vi "add units.vi"(7 "Language":string, 9 "Array":dbl[](array[numeric]), 10 "Numeric":dbl, 11 "Label Text":string) -> (1 "Converted Array":dbl[](array[numeric]), 2 "Converted Numeric":dbl, 3 "unit in brackets":string, 4 "format string":string, 5 "unit":string)   [LabVIEW 2015]
panel:
  # "Et\tEntrance Tank\tformerly grit chamber\nAmp\tamplitude\tL\nB\tperpendicular distance between components (center to center)\tL\nE\tpipe roughness\tL\nFB\tFreeboard\tL\nH\theight (includes freeboard)\tL\nHL\thead loss\tL\nHW\tlocal water depth\tL\nID\tinner diameter\tL\nL\tlength\tL\nLoc\tLocations\tL\nND\tnominal diameter\tL\nOD\touter diameter\tL\nR\tRadius\tL\nS\tspace between components\tL\nT\tthickness\tL\nW\twidth\tL\nZ\televation relative to bottom of sed tank\tL\nZW\twater depth relative to bottom of sed tank\tL\nV\tvelocity\tL/T\nCP\tCollision Potential\tL^(2/3)\nA\tArea\tL^2\nNu\tkinematic viscosity\tL^2/T\nED\tenergy dissipation rate\tL^2/T^3\nVol\tvolume\tL^3\nQ\tflow\tL^3/T\nMW\tMolecular weight\tM\nC\tConcentration\tM/L^3\nRho\tDensity\tM/L^3\nAN\tangle\tradians\nTi\ttime\tT"
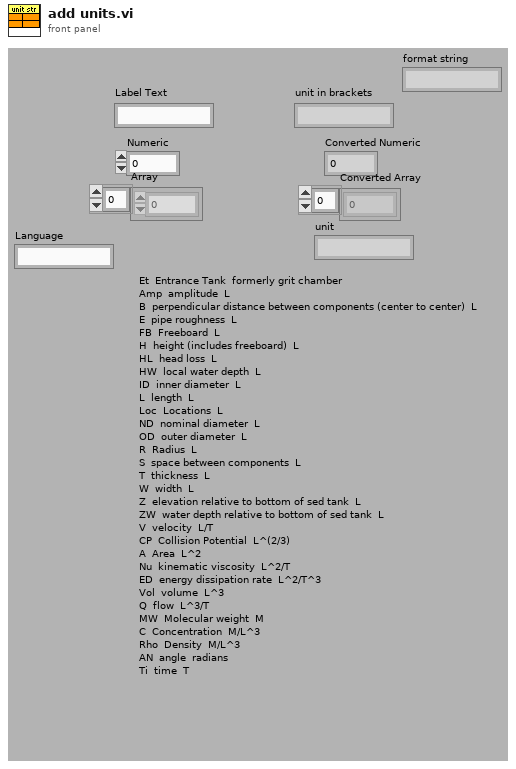
[diagram p1: front panel]
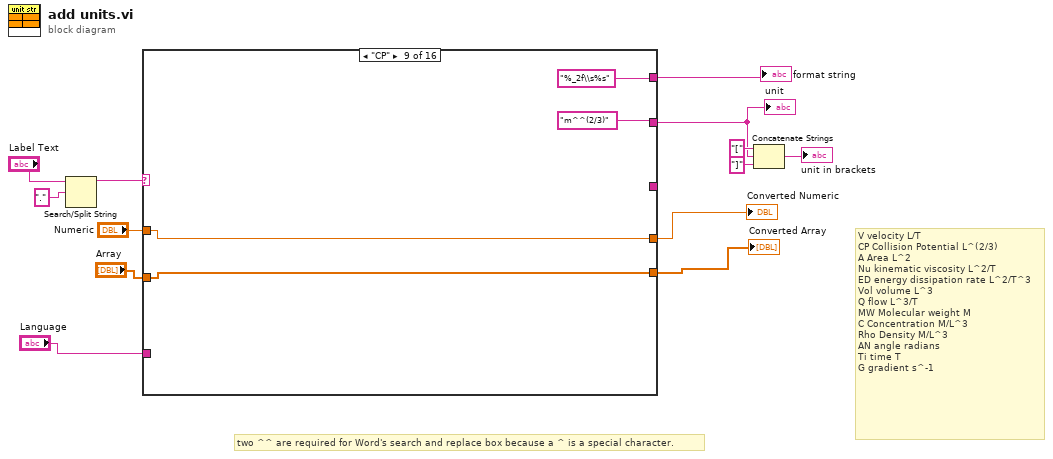
[diagram p0: block diagram]
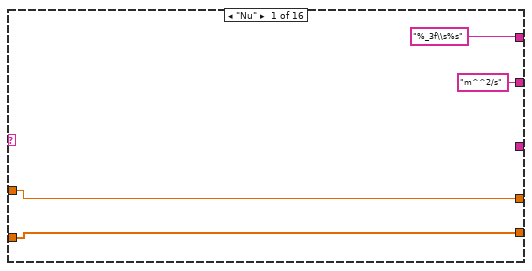
[diagram p2: hidden frame]
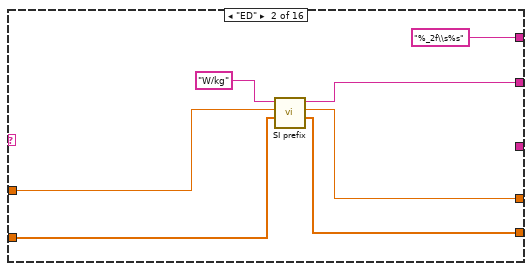
[diagram p3: hidden frame]
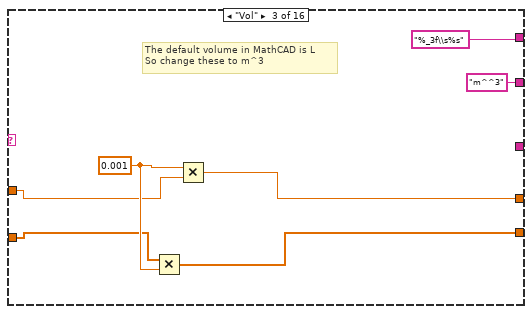
[diagram p4: hidden frame]
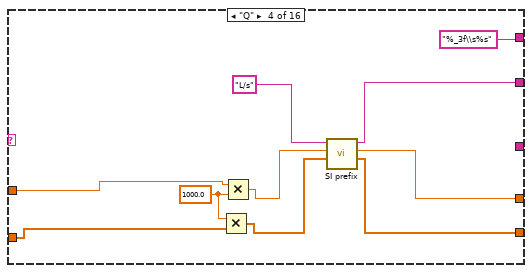
[diagram p5: hidden frame]
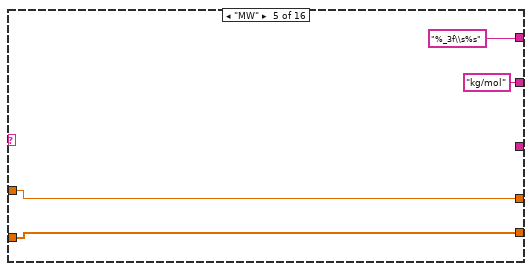
[diagram p6: hidden frame]
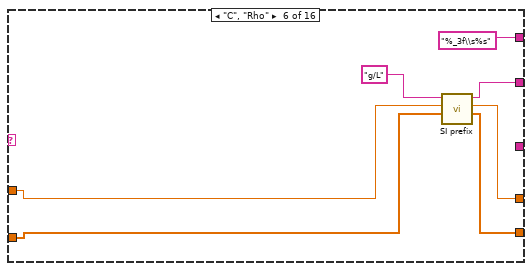
[diagram p7: hidden frame]
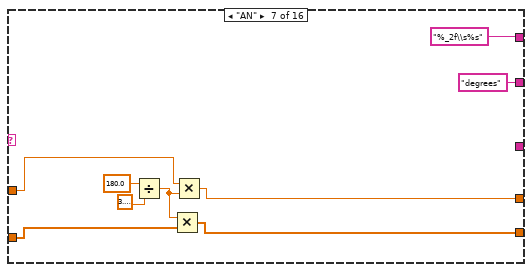
[diagram p8: hidden frame]
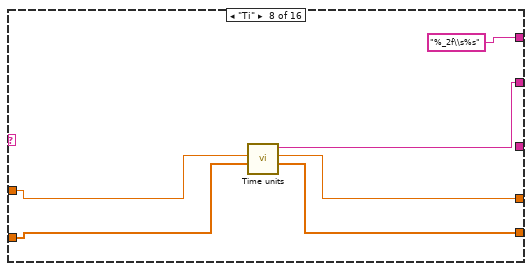
[diagram p9: hidden frame]
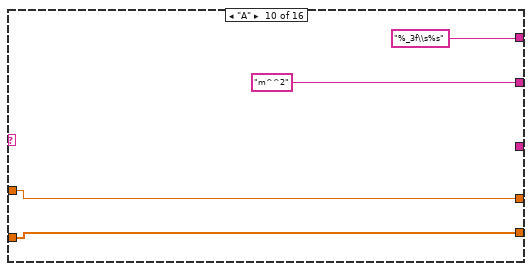
[diagram p10: hidden frame]
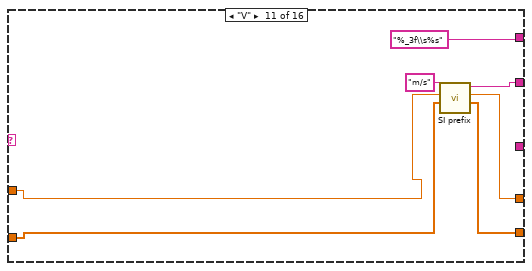
[diagram p11: hidden frame]
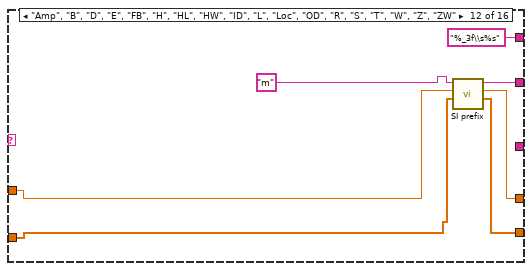
[diagram p12: hidden frame]
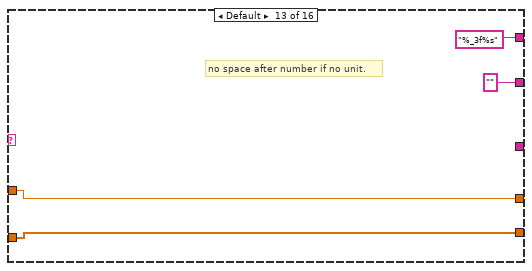
[diagram p13: hidden frame]
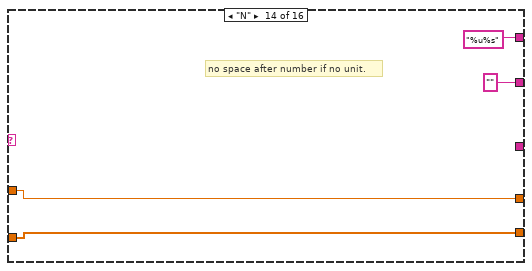
[diagram p14: hidden frame]
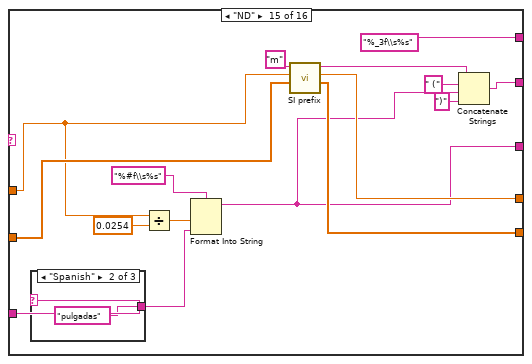
[diagram p15: hidden frame]
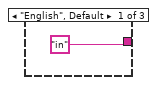
[diagram p16: hidden frame]
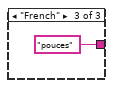
[diagram p17: hidden frame]
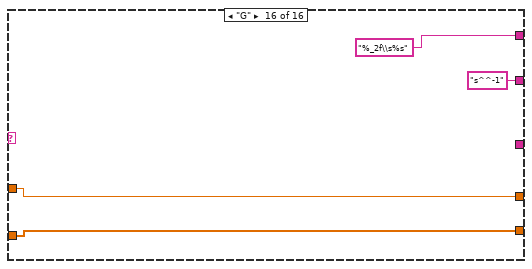
[diagram p18: hidden frame]
diagram:
  # "two ^^ are required for Word's search and replace box because a ^ is a special character."
  # "V\tvelocity\tL/T\nCP\tCollision Potential\tL^(2/3)\nA\tArea\tL^2\nNu\tkinematic viscosity\tL^2/T\nED\tenergy dissipation rate\tL^2/T^3\nVol\tvolume\tL^3\nQ\tflow\tL^3/T\nMW\tMolecular weight\tM\nC\tConcentration\tM/L^3\nRho\tDensity\tM/L^3\nAN\tangle\tradians\nTi\ttime\tT\nG gradient s^-1"
  n1 = Search/Split String(string="Label Text", search string/char (-)="." ("regular expression")) -> (substring before match=w11:string)  [unwired: 1 in, 2 out]
  n2 = case shown="\"CP\"" w11 {
    tunnel: ["m^^2/s" w22 "m^^3" w36 "kg/mol" w50 "degrees" w62 "m^^(2/3)" "m^^2" w80 w87 "" "" w103 "s^^-1" ("modified unit")] -> w4
    tunnel: "Numeric" -> [w16 w21 w28 w40 w44 w49 w57 w66 w70 w74 w77 w86 w92 w96 w109 w119]
    tunnel: "Array" -> [w15 w20 w26 w39 w43 w47 w56 w65 w69 w73 w79 w84 w91 w95 w112 w118]
    tunnel: [w15 w18 w25 w32 w43 w46 w54 w64 w69 w73 w78 w83 w91 w95 w111 w118] -> w2
    tunnel: [w16 w19 w27 w34 w44 w48 w55 w63 w70 w74 w76 w85 w92 w96 w110 w119] -> w3
    tunnel: ["%_3f\\s%s" "%_2f\\s%s" "%_3f\\s%s" "%_3f\\s%s" "%_3f\\s%s" "%_3f\\s%s" "%_2f\\s%s" "%_2f\\s%s" "%_2f\\s%s" "%_3f\\s%s" "%_3f\\s%s" "%_3f\\s%s" "%_3f%s" "%u%s" "%_3f\\s%s" "%_2f\\s%s"] -> w5
    tunnel: [_ _ _ _ _ _ _ _ _ _ _ _ _ _ w102 _] -> _
    tunnel: "Language" -> [_ _ _ _ _ _ _ _ _ _ _ _ _ _ w99 _]
    frame "Nu" {
    }
    frame "ED" {
      n3 = call "SI prefix.vi"("Array"=w20, "Numeric"=w21, "Unit"="W/kg") -> ("Scaled Array"=w18:dbl[], "Scaled Number"=w19:dbl, "modified unit"=w22:string)  [unwired: 6 in]
    }
    frame "Vol" {
      w29 = 0.001 ("x")
      # "The default volume in MathCAD is L\nSo change these to m^3"
      n4 = Multiply(x=w26, y=w29) -> (x*y=w25:dbl[])
      n5 = Multiply(x=w29, y=w28) -> (x*y=w27:dbl)
    }
    frame "Q" {
      w41 = 1000.0 ("y")
      n6 = Multiply(x=w41, y=w39) -> (x*y=w33:dbl[])
      n7 = Multiply(x=w40, y=w41) -> (x*y=w35:dbl)
      n8 = call "SI prefix.vi"("Array"=w33, "Numeric"=w35, "Unit"="L/s") -> ("Scaled Array"=w32:dbl[], "Scaled Number"=w34:dbl, "modified unit"=w36:string)  [unwired: 6 in]
    }
    frame "MW" {
    }
    frame "C", "Rho" {
      n9 = call "SI prefix.vi"("Array"=w47, "Numeric"=w49, "Unit"="g/L") -> ("Scaled Array"=w46:dbl[], "Scaled Number"=w48:dbl, "modified unit"=w50:string)  [unwired: 6 in]
    }
    frame "AN" {
      n10 = Divide(x=180.0 ("y"), y=3.141592653589793) -> (x/y=w60:dbl)
      n11 = Multiply(x=w60, y=w56) -> (x*y=w54:dbl[])
      n12 = Multiply(x=w57, y=w60) -> (x*y=w55:dbl)
    }
    frame "Ti" {
      n13 = call "Time units.vi"("Array"=w65, "Numeric"=w66) -> ("Scaled Array"=w64:dbl[], "Scaled Number"=w63:dbl, "modified unit"=w62:string)  [unwired: 7 in]
    }
    frame "CP" {
    }
    frame "A" {
    }
    frame "V" {
      n14 = call "SI prefix.vi"("Array"=w79, "Numeric"=w77, "Unit"="m/s") -> ("Scaled Array"=w78:dbl[], "Scaled Number"=w76:dbl, "modified unit"=w80:string)  [unwired: 6 in]
    }
    frame "Amp", "B", "D", "E", "FB", "H", "HL", "HW", "ID", "L", "Loc", "OD", "R", "S", "T", "W", "Z", "ZW" {
      n15 = call "SI prefix.vi"("Array"=w84, "Numeric"=w86, "Unit"="m") -> ("Scaled Array"=w83:dbl[], "Scaled Number"=w85:dbl, "modified unit"=w87:string)  [unwired: 6 in]
    }
    frame Default {
      # "no space after number if no unit."
    }
    frame "N" {
      # "no space after number if no unit."
    }
    frame "ND" {
      n16 = case shown="\"Spanish\"" w99 {
        tunnel: ["in" ("input 2") "pulgadas" "pouces"] -> w98
        frame "English", Default {
        }
        frame "Spanish" {
        }
        frame "French" {
        }
      }
      n17 = Divide(x=w109, y=0.0254) -> (x/y=w107:dbl)
      n18 = Format Into String(format string="%#f\\s%s", w107, w98) -> (resulting string=w102:string)  [unwired: 2 in, 1 out]
      n19 = call "SI prefix.vi"("Array"=w112, "Numeric"=w109, "Unit"="m") -> ("Scaled Array"=w111:dbl[], "Scaled Number"=w110:dbl, "modified unit"=w104:string)  [unwired: 6 in]
      n20 = Concatenate Strings(w104, " (" ("string"), w102, ")" ("string")) -> (w103:string)
    }
    frame "G" {
    }
  }
  "Converted Numeric" <- w3
  "Converted Array" <- w2
  "unit" <- w4
  "format string" <- w5
  n21 = Concatenate Strings("[" ("string"), w4, "]" ("string")) -> (→"unit in brackets":string)
